vi "DHE_SetExpOverhead.vi"(10 "ExpOverhead":string) -> ()   [LabVIEW 2016]
uses:
  private/vis/DHE_VarAction.ctl
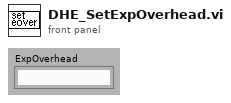
[diagram p1: front panel]
types:
  T1 = typedef "DHE_VarAction.ctl" = enum16{"read", "write"}
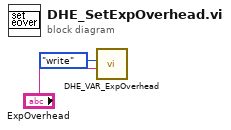
[diagram p0: block diagram]
diagram:
  n1 = call "DHE_VAR_ExpOverhead.vi"("value"="ExpOverhead", "action"=DHE_VarAction."write") -> ()  [unwired: 10 out]
